vi "SRX_Config_Set Output Values.vi"(6 "Send Cmd Timout(ms)":u32, 8 "Error":errorcluster, 9 "SRX Output":T1={"Neutral"=enum."Override to Coast", "Max"={"FWD"=1.0, "REV"=-1.0}, "Min"={"FWD"=1.0, "REV"=-1.0}, "OL Ramp Rate (S)"=0.0, "Dead Band"=0.0, "CL Ramp Rate (S)"=0.0} {"Min"."REV" format="%.2f"; "Min"."FWD" format="%.2f"; "Max"."REV" format="%.2f"; "Max"."FWD" format="%.2f"}, 11 "PhoenixMotorControlDevRef":T4) -> (0 "Error Out":errorcluster, 3 "PhoenixMotorControlDevRef Out":T4)   [LabVIEW 2023]
uses:
  <vilib>/Rock Robotics/WPI/MotorControl/WPI_MotorControlDeviceRef.ctl
  <vilib>/Rock Robotics/WPI/MotorControl/WPI_MotorControlType.ctl
  <vilib>/Rock Robotics/SystemInterfaces/DIO/FPGA_DIOPWMChannel.ctl
  <vilib>/Rock Robotics/WPI/PWM/WPI_PWMDeadband.ctl
  <vilib>/Rock Robotics/SystemInterfaces/DIO/FPGA_DIOChannel.ctl
  Shared Code/TypeDefs/Cluster_Config SRX Motor Output.ctl
  <vilib>/Rock Robotics/WPI/ThirdParty/Phoenix-LabVIEW/Motor Controller/Controls/CTRE_Phoenix_MotorControl_NeutralMode.ctl
  Shared Code/TypeDefs/Cluster_FWD  REV Values.ctl
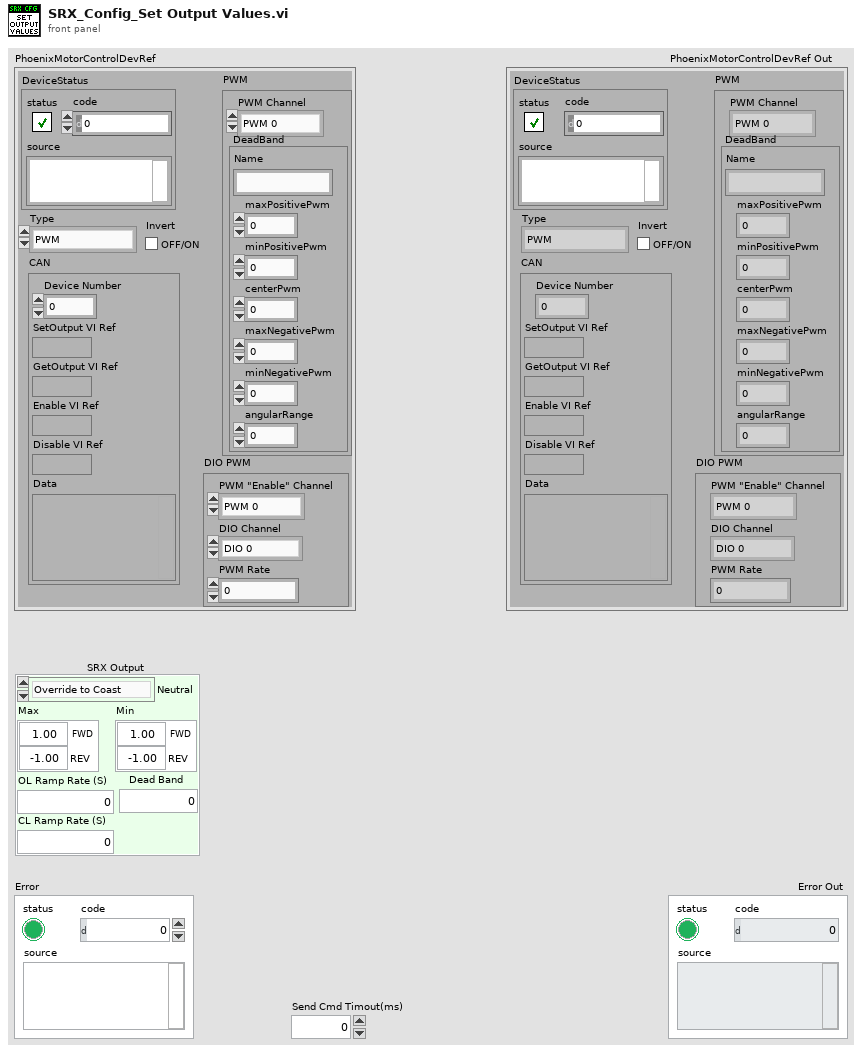
[diagram p1: front panel]
types:
  T1 = typedef "Cluster_Config SRX Motor Output.ctl" = cluster{"Neutral":T2, "Max":T3, "Min":T3, "OL Ramp Rate (S)":dbl, "Dead Band":dbl, "CL Ramp Rate (S)":dbl}
  T2 = typedef "CTRE_Phoenix_MotorControl_NeutralMode.ctl" = enum8{"EEPROMSetting", "Override to Coast", "Override to Brake"}
  T3 = typedef "Cluster_FWD  REV Values.ctl" = cluster{"FWD":dbl, "REV":dbl}
  T4 = typedef "WPI_MotorControlDeviceRef.ctl" = cluster{"DeviceStatus":errorcluster, "Type":T5, "PWM":cluster{"PWM Channel":T6, "DeadBand":T7}, "CAN":cluster{"Device Number":u8, "SetOutput VI Ref":variant, "GetOutput VI Ref":variant, "Enable VI Ref":variant, "Disable VI Ref":variant, "Data":variant}, "Invert":bool, "DIO PWM":cluster{"PWM \"Enable\" Channel":T6, "DIOChannel":T8, "PWM Rate":dbl}}
  T5 = typedef "WPI_MotorControlType.ctl" = enum16{"PWM", "CAN", "DIO PWM"}
  T6 = typedef "FPGA_DIOPWMChannel.ctl" = enum8{"PWM 0", "PWM 1", "PWM 2", "PWM 3", "PWM 4", "PWM 5", "PWM 6", "PWM 7", "PWM 8", "PWM 9", "PWM MXP 0", "PWM MXP 1", "PWM MXP 2", "PWM MXP 3", "PWM MXP 4", "PWM MXP 5", "PWM MXP 6", "PWM MXP 7", "PWM MXP 8", "PWM MXP 9", "Invalid"}
  T7 = typedef "WPI_PWMDeadband.ctl" = cluster{"Name":string, "maxPositivePwm":i32, "minPositivePwm":i32, "centerPwm":i32, "maxNegativePwm":i32, "minNegativePwm":i32, "angularRange":u16}
  T8 = typedef "FPGA_DIOChannel.ctl" = enum8{"DIO 0", "DIO 1", "DIO 2", "DIO 3", "DIO 4", "DIO 5", "DIO 6", "DIO 7", "DIO 8", "DIO 9", "DIO MXP 0", "DIO MXP 1", "DIO MXP 2", "DIO MXP 3", "DIO MXP 4", "DIO MXP 5", "DIO MXP 6", "DIO MXP 7", "DIO MXP 8", "DIO MXP 9", "DIO MXP 10", "DIO MXP 11", "DIO MXP 12", "DIO MXP 13", "DIO MXP 14", "DIO MXP 15", "SPI Port CS1", "SPI Port CS2", "SPI Port CS3", "SPI Port MISO", "SPI Port MOSI", "Invalid"}
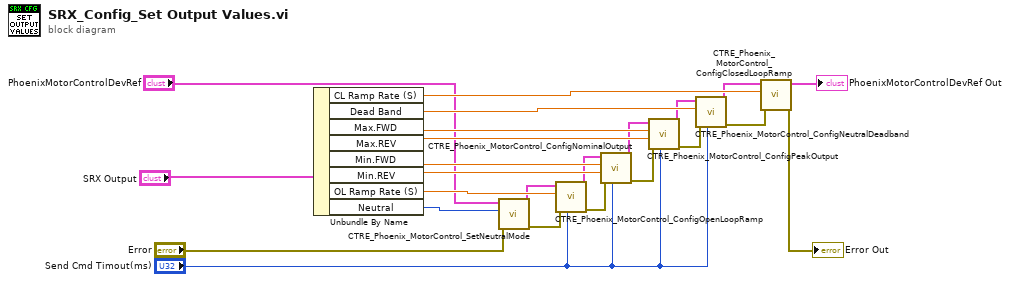
[diagram p0: block diagram]
diagram:
  n1 = Unbundle By Name("SRX Output") -> ("CL Ramp Rate (S)"=w6:dbl, "Dead Band"=w9:dbl, "Max.FWD"=w12:dbl, "Max.REV"=w13:dbl, "Min.FWD"=w16:dbl, "Min.REV"=w17:dbl, "OL Ramp Rate (S)"=w20:dbl, "Neutral"=w21:T2)
  n2 = call <vilib>:"CTRE_Phoenix_MotorControl_SetNeutralMode.vi"("error in (no error)"="Error", "Motor Control Neutral Mode"=w21, "PhoenixMotorControlDevRef"="PhoenixMotorControlDevRef") -> ("error out"=w18:errorcluster, "PhoenixMotorControlDevRef"=w19:T4)  [unwired: 7 in]
  n3 = call <vilib>:"CTRE_Phoenix_MotorControl_ConfigOpenLoopRamp.vi"("timeoutMs"="Send Cmd Timout(ms)", "error in (no error)"=w18, "secondsFromNeutralToFull"=w20, "PhoenixMotorControlDevRef"=w19) -> ("error out"=w14:errorcluster, "PhoenixMotorControlDevRef"=w15:T4)  [unwired: 6 in]
  n4 = call <vilib>:"CTRE_Phoenix_MotorControl_ConfigNominalOutput.vi"("timeoutMs"="Send Cmd Timout(ms)", "error in (no error)"=w14, "Reverse Nominal Percent Output"=w17, "Forward Nominal Percent Output"=w16, "PhoenixMotorControlDevRef"=w15) -> ("error out"=w10:errorcluster, "PhoenixMotorControlDevRef"=w11:T4)  [unwired: 5 in]
  n5 = call <vilib>:"CTRE_Phoenix_MotorControl_ConfigPeakOutput.vi"("timeoutMs"="Send Cmd Timout(ms)", "error in (no error)"=w10, "Reverse Peak Percent Output"=w13, "Forward Peak Percent Output"=w12, "PhoenixMotorControlDevRef"=w11) -> ("error out"=w7:errorcluster, "PhoenixMotorControlDevRef"=w8:T4)  [unwired: 5 in]
  n6 = call <vilib>:"CTRE_Phoenix_MotorControl_ConfigNeutralDeadband.vi"("timeoutMs"="Send Cmd Timout(ms)", "error in (no error)"=w7, "Percent Deadband"=w9, "PhoenixMotorControlDevRef"=w8) -> ("error out"=w4:errorcluster, "PhoenixMotorControlDevRef"=w5:T4)  [unwired: 6 in]
  n7 = call <vilib>:"CTRE_Phoenix_MotorControl_ConfigClosedLoopRamp.vi"("error in (no error)"=w4, "secondsFromNeutralToFull"=w6, "PhoenixMotorControlDevRef"=w5) -> ("error out"=→"Error Out":errorcluster, "PhoenixMotorControlDevRef"=→"PhoenixMotorControlDevRef Out":T4)  [unwired: 7 in]
